vi "svl_Check Data Valid (N Ch) [SLM].vi"(4 "decimation factor":i32=1 min=1 step=1, 5 "time constant [ms]":dbl=125.0 format="%.2f", 6 "integration time [s]":dbl=1.0 format="%.2f", 7 "exponential mode":enum16{"Slow", "Fast", "Impulse", "Custom"}(ring)=enum."Fast", 8 "error in (no error)":errorcluster, 9 "restart averaging (F)":bool, 10 "level analysis":T2(ring), 11 "scaled signals [EU]":waveform(dbl)[](array[waveform])) -> (0 "error out":errorcluster, 1 "processing state":T1(ring), 3 "dup scaled signals [EU]":waveform(dbl)[](array[waveform]))   [LabVIEW 2017]
uses:
  <vilib>/addons/_NISVFA/_Shared subVIs/Common/svc_Check for Waveform Parameter Continuity (no state).vi
  <vilib>/addons/_NISVFA/_Shared subVIs/Common/svc_Get SV Channel Info.vi
  <vilib>/addons/_NISVFA/_Shared subVIs/Common/svc_Engineering Units to Unit Label.vi
  <vilib>/addons/_NISVFA/_Shared subVIs/Common/svc_Unit Label to Engineering Units.vi
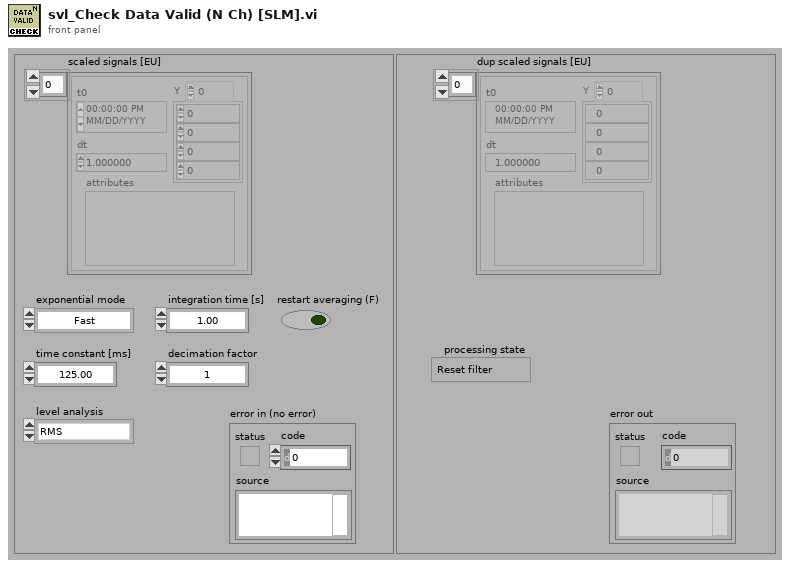
[diagram p1: front panel]
types:
  T1 = enum16{"Reset filter", "Restart averaging", "Continue processing"}
  T2 = enum16{"RMS", "Running RMS", "Exp avg  ", "Dec exp avg ", "Peak", "Crest"}
  T3 = cluster{"dt":bool, "t0 continuity":bool, "array length":bool, "channel info":bool, "name":bool}
  T4 = cluster{"dt equal":bool, "array length equal":bool, "number channels change":bool}
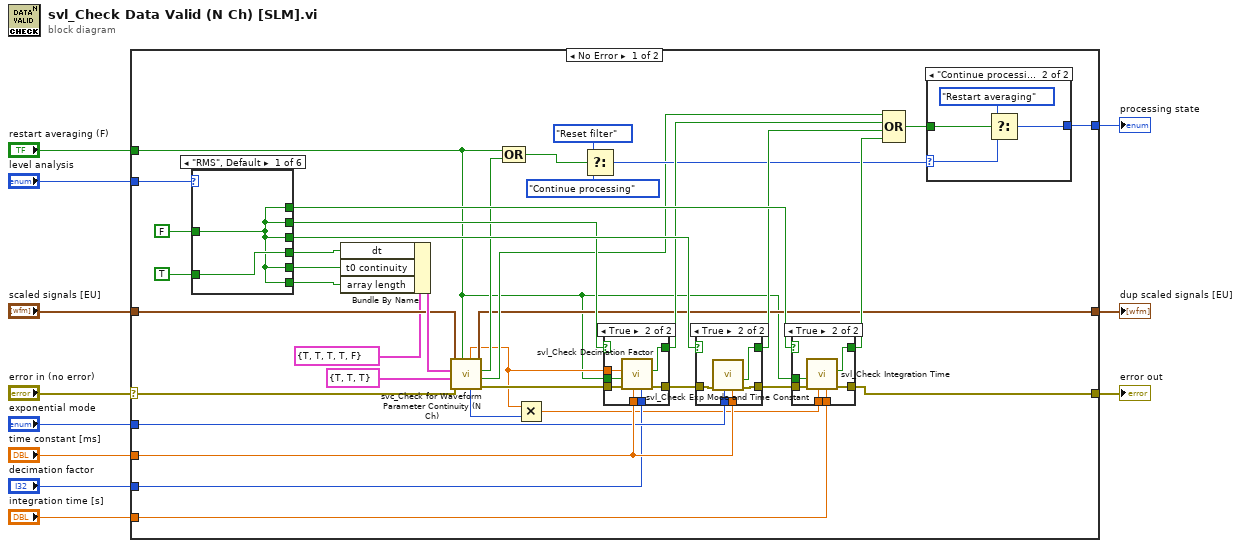
[diagram p0: block diagram]
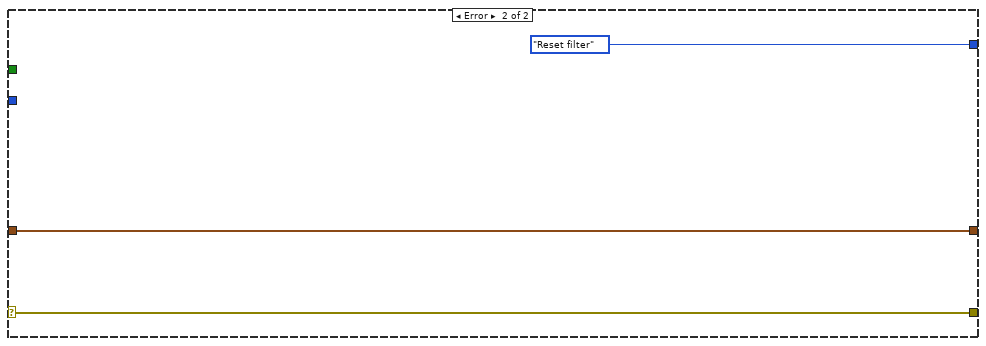
[diagram p11: hidden frame]
diagram:
  n1 = case shown="No Error" "error in (no error)" {
    selector: "error in (no error)" -> [w24 w92]
    tunnel: [w23 w92] -> w10
    tunnel: "scaled signals [EU]" -> [w29 w90]
    tunnel: "restart averaging (F)" -> [w14 _]
    tunnel: "time constant [ms]" -> [w28 _]
    tunnel: [w49 T1."Reset filter" ("processing state")] -> w7
    tunnel: "level analysis" -> [w30 _]
    tunnel: "integration time [s]" -> [w25 _]
    tunnel: "decimation factor" -> [w26 _]
    tunnel: "exponential mode" -> [w27 _]
    tunnel: [w18 w90] -> w1
    frame No Error {
      n2 = case shown="\"RMS\", Default" w30 {
        tunnel: [w74 w77 w79 w81 w82 w83] -> w45
        tunnel: [w74 w77 w78 w81 w82 w83] -> w44
        tunnel: [w74 w76 w78 w80 w82 w83] -> w43
        tunnel: [w74 w76 w78 w80 w82 w83] -> w31
        tunnel: [w74 w76 w79 w81 w82 w83] -> w40
        tunnel: [w75 w76 w79 w81 w82 w84] -> w39
        tunnel: FALSE -> [w74 w77 w78 w80 w82 w83]
        tunnel: TRUE -> [w75 w76 w79 w81 _ w84]
        frame "RMS", Default {
        }
        frame "Running RMS" {
        }
        frame "Exp avg  " {
        }
        frame "Dec exp avg " {
        }
        frame "Peak" {
        }
        frame "Crest" {
        }
      }
      n3 = Bundle By Name(cluster=T3 {"dt"=TRUE, "t0 continuity"=TRUE, "array length"=TRUE, "channel info"=TRUE, "name"=FALSE} ("checks for channel parameter change"), "dt"=w39, "t0 continuity"=w40, "array length"=w31) -> (w41:T3)
      n4 = call <vilib>:"svc_Check for Waveform Parameter Continuity (N Ch).vi"("restart averaging (F)"=w14, "error in (no error)"=w24, "checks for multichannel parameters"=T4 {"dt equal"=TRUE, "array length equal"=TRUE, "number channels change"=TRUE}, "checks for channel parameter change"=w41, "scaled signal(s)"=w29) -> ("error out"=w36:errorcluster, "multichannel parameter changed"=w19:bool, "waveform parameter changed"=w20:bool, "dup scaled signal(s)"=w18:waveform(dbl)[], "array length"=w16:i32, "dt"=w17:dbl)  [unwired: 1 out]
      n5 = Compound Arithmetic op=OR(w14, w20) -> (w42:bool)
      n6 = Multiply(x=w17, y=w16) -> (x*y=w15:dbl)
      n7 = Select(t=T1."Reset filter" ("processing state"), s=w42, f=T1."Continue processing" ("processing state")) -> (s? t:f=w22:T1)
      n8 = case shown="True" w44 {
        selector: w44 -> [w58 _]
        tunnel: w36 -> [w59 w66]
        tunnel: [w59 w65] -> w38
        tunnel: w28 -> [_ w64]
        tunnel: w26 -> [_ w63]
        tunnel: [w58 w61] -> w34
        tunnel: w17 -> [_ w62]
        tunnel: w14 -> [_ w60]
        frame False {
        }
        frame True {
          n9 = call <vilib>:"svl_Check Decimation Factor.vi"("decimation factor"=w63, "time constant [ms]"=w64, "error in (no error)"=w66, "restart averaging (F)"=w60, "dt"=w62) -> ("error out"=w65:errorcluster, "parameter has changed"=w61:bool)  [unwired: 5 in]
        }
      }
      n10 = case shown="True" w45 {
        selector: w45 -> [w67 _]
        tunnel: w27 -> [_ w73]
        tunnel: w38 -> [w68 w69]
        tunnel: [w68 w72] -> w37
        tunnel: [w67 w70] -> w35
        tunnel: w28 -> [_ w71]
        frame False {
        }
        frame True {
          n11 = call <vilib>:"svl_Check Exp Mode and Time Constant.vi"("time constant [ms]"=w71, "exponential mode"=w73, "error in (no error)"=w69) -> ("error out"=w72:errorcluster, "parameter has changed"=w70:bool)  [unwired: 7 in]
        }
      }
      n12 = case shown="True" w43 {
        selector: w43 -> [w50 _]
        tunnel: w37 -> [w51 w57]
        tunnel: [w51 w56] -> w23
        tunnel: w25 -> [_ w54]
        tunnel: [w50 w55] -> w48
        tunnel: w15 -> [_ w53]
        tunnel: w14 -> [_ w52]
        frame False {
        }
        frame True {
          n13 = call <vilib>:"svl_Check Integration Time.vi"("integration time"=w54, "acquisition period"=w53, "error in (no error)"=w57, "restart averaging (F)"=w52) -> ("error out"=w56:errorcluster, "parameter has changed"=w55:bool)  [unwired: 5 in, 1 out]
        }
      }
      n14 = Compound Arithmetic op=OR(w19, w34, w35, w48) -> (w21:bool)
      n15 = case shown="\"Continue processing\"" w22 {
        selector: w22 -> [w85 w88]
        tunnel: w21 -> [_ w89]
        tunnel: [w85 w86] -> w49
        frame "Reset filter", Default {
        }
        frame "Continue processing" {
          n16 = Select(t=T1."Restart averaging" ("processing state"), s=w89, f=w88) -> (s? t:f=w86:T1)
        }
      }
    }
    frame Error {
      (unwired) TRUE ("t0 changed")
    }
  }
  "error out" <- w10
  "processing state" <- w7
  "dup scaled signals [EU]" <- w1
